vi "ErrorHandler.vi"(8 "error in (no error)":errorcluster, 11 "Queue in":refnum<queue>) -> (0 "error out":errorcluster, 3 "Queue out":refnum<queue>)   [LabVIEW 2019]
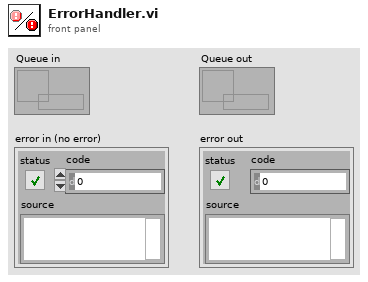
[diagram p1: front panel]
types:
  T1 = cluster{"Consumer State":string, "Received Data":string, "error constant":errorcluster}
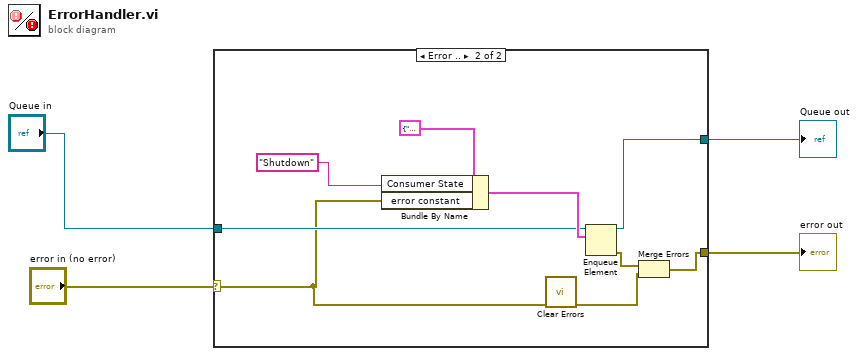
[diagram p0: block diagram]
diagram:
  n1 = case shown="Error .." "error in (no error)" {
    selector: "error in (no error)" -> [w5 w8]
    tunnel: "Queue in" -> [w6 w12]
    tunnel: [w6 w11] -> w3
    tunnel: [w5 w9] -> w4
    frame No Error {
    }
    frame Error {
      n2 = Bundle By Name(cluster=T1 {"Consumer State"="Default", "Received Data"="", "error constant"={"status"=FALSE, "code"=0, "source"=""}} ("Cluster 2"), "Consumer State"="Shutdown", "error constant"=w8) -> (w13:T1)
      n3 = call <vilib>:"Clear Errors.vi"("error in (no error)"=w8) -> ("error out"=w7:errorcluster)  [unwired: 5 in, 1 out]
      n4 = Enqueue Element(queue=w12, element=w13) -> (queue out=w11:refnum<queue>, error out=w10:errorcluster)  [unwired: 2 in, 1 out]
      n5 = Merge Errors(w10, w7) -> (w9:errorcluster)
    }
  }
  "error out" <- w4
  "Queue out" <- w3
